vi "Inst_CNT90.vi"(8 "error in":errorcluster, 10 "All Message Queues in":T1, 11 "Prueba31 in":refnum<class "Prueba06.lvclass">) -> (0 "error out":errorcluster)   [LabVIEW 2019, in "Prueba06.lvclass"]
uses:
  Prueba06.lvclass
  QMH/Message Queue/All Message Queues.ctl
  QMH/Message Queue/Message Cluster.ctl
  Prueba06.lvclass/Prueba06.ctl
  <vilib>/Utility/error.llb/Error Cluster From Error Code.vi
  QMH/Message Queue/Enqueue Message (Single).vi
  <vilib>/ErrorRing/Error Ring.xnode
  QMH/Message Queue/Message Queue.lvlib
  Instrumento/CNT90/CNT90.lvclass
panel:
  out "All States":string[](array[string])
  out "Actual State":string
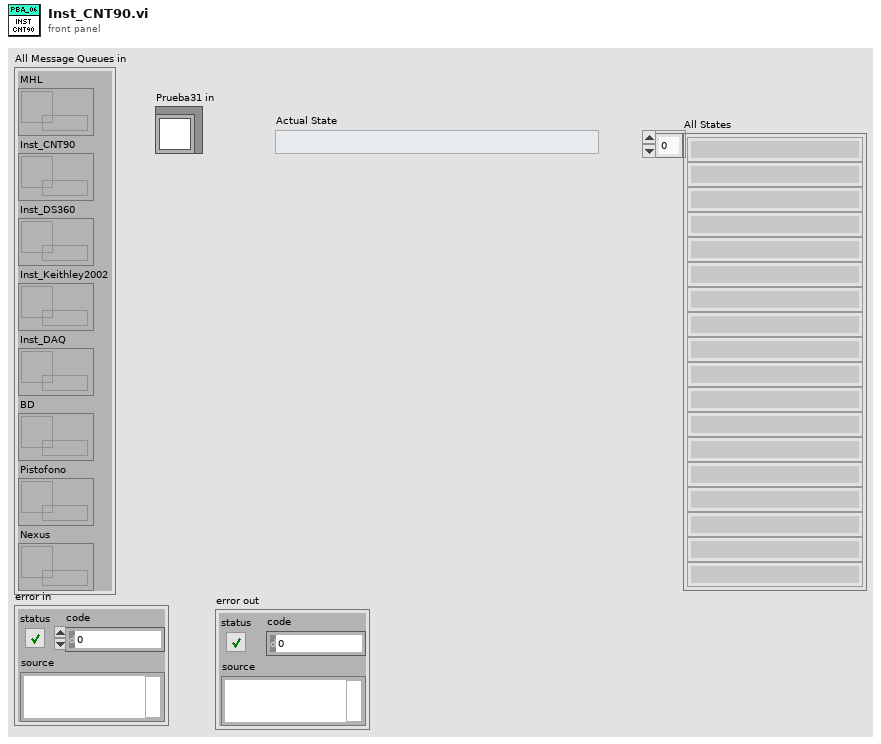
[diagram p1: front panel]
types:
  T1 = typedef "Message Queue.lvlib/All Message Queues.ctl" = cluster{"MHL":refnum<queue>, "Inst_CNT90":refnum<queue>, "Inst_DS360":refnum<queue>, "Inst_Keithley2002":refnum<queue>, "Inst_DAQ":refnum<queue>, "BD":refnum<queue>, "Pistofono":refnum<queue>, "Nexus":refnum<queue>}
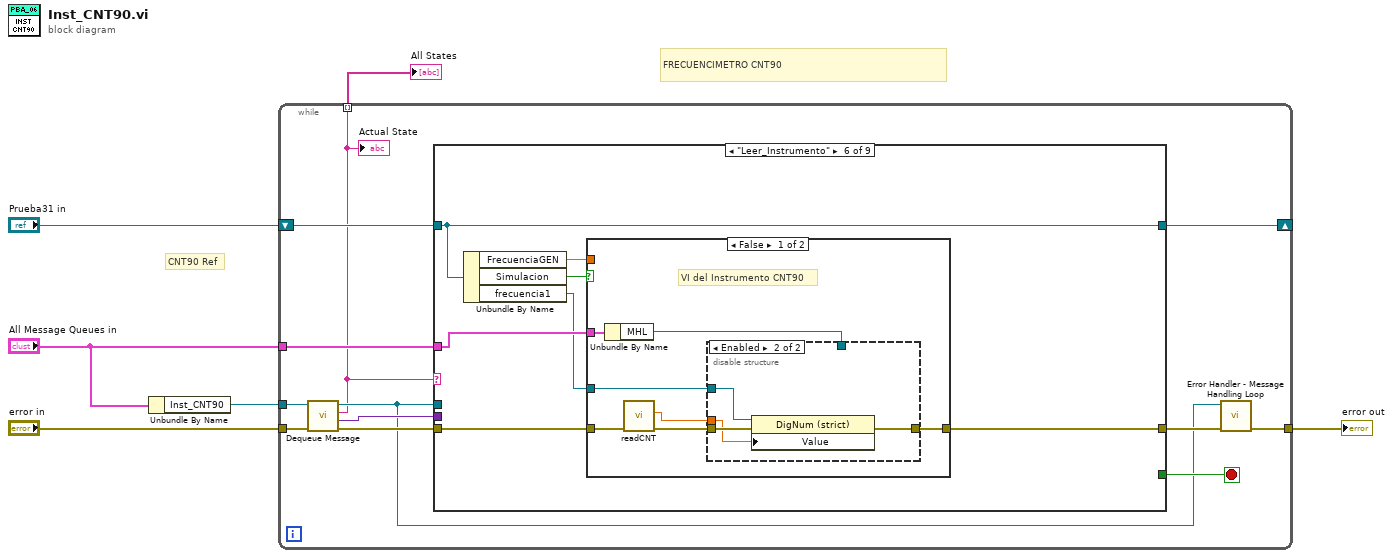
[diagram p0: block diagram]
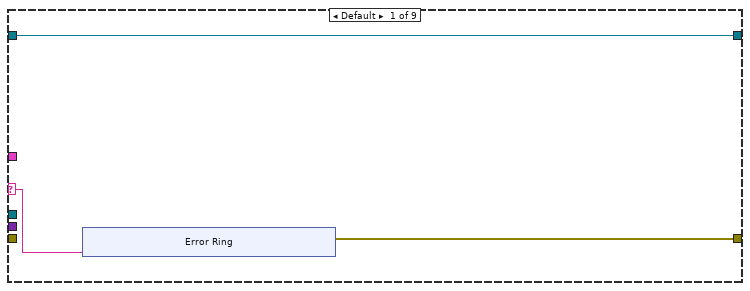
[diagram p2: hidden frame]
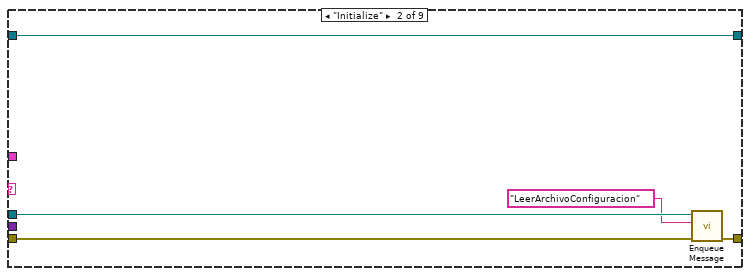
[diagram p3: hidden frame]
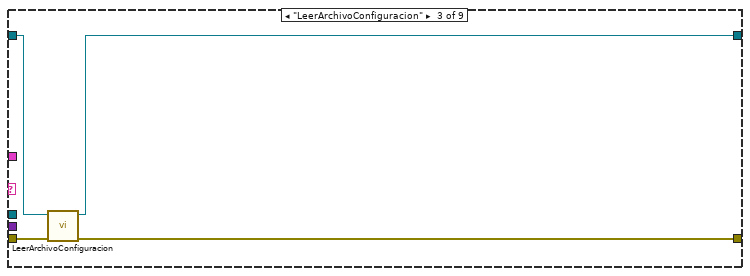
[diagram p4: hidden frame]
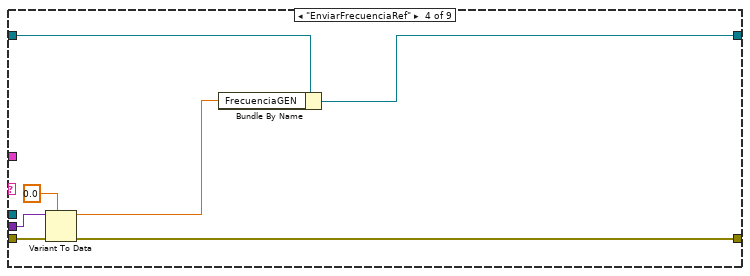
[diagram p5: hidden frame]
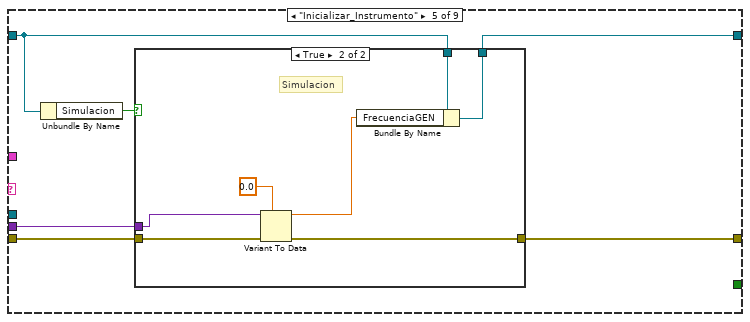
[diagram p6: hidden frame]
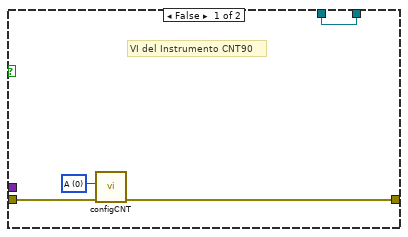
[diagram p7: hidden frame]
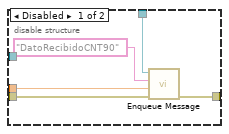
[diagram p8: hidden frame]
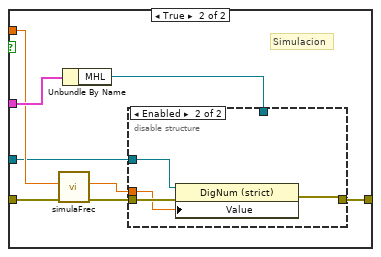
[diagram p9: hidden frame]
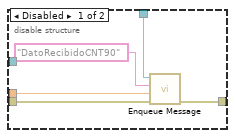
[diagram p10: hidden frame]
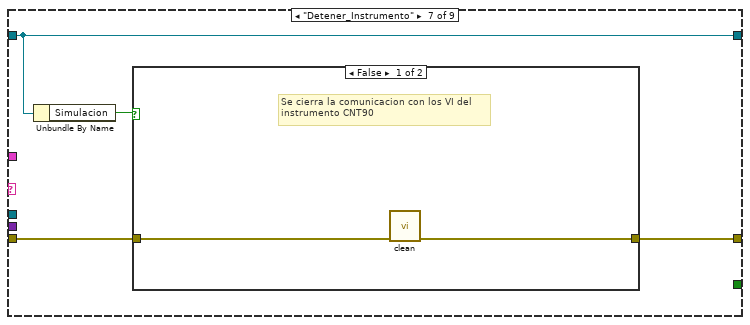
[diagram p11: hidden frame]
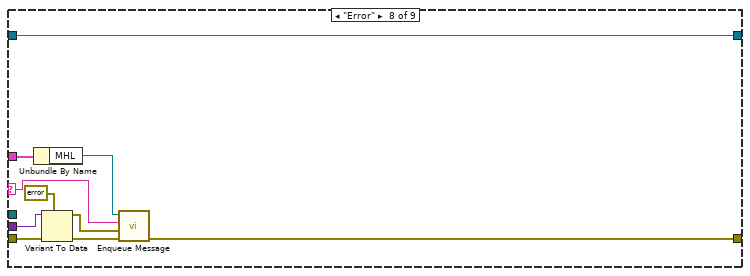
[diagram p13: hidden frame]
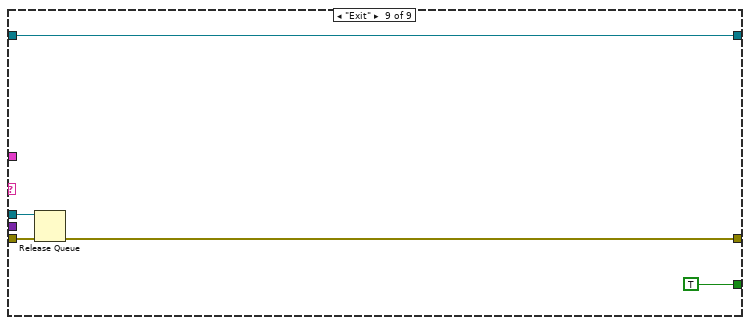
[diagram p14: hidden frame]
diagram:
  # "FRECUENCIMETRO CNT90"
  # "CNT90 Ref"
  n1 = Unbundle By Name("All Message Queues in") -> ("Inst_CNT90"=w4:refnum<queue>)
  n2 = while {
    tunnel: "error in" -> [w18]
    tunnel: w4 -> [w17]
    tunnel: "All Message Queues in" -> [w16]
    tunnel: [w9] -> w2
    shift-right: [w12] -> _
    shift-left: "Prueba31 in" -> [w15]
    tunnel: [w7] -> w1 mode=indexing
    stop <- w11 stop-if-true
    n3 = call "Dequeue Message.vi"("error in (no error)"=w18, "Message Queue"=w17) -> ("error out"=w13:errorcluster, "Message Data"=w14:variant, "Message"=w7:string, "dup Message Queue"=w8:refnum<queue>)  [unwired: 6 in]
    "Actual State" <- w7
    n4 = case shown="\"Leer_Instrumento\"" w7 {
      selector: w7 -> [w21 _ _ _ _ _ _ w113 _]
      tunnel: w16 -> [_ _ _ _ _ w64 _ w112 _]
      tunnel: w15 -> [w19 w33 w34 w39 w46 w66 w104 w110 w120]
      tunnel: w8 -> [_ w30 _ _ _ _ _ _ w122]
      tunnel: w14 -> [_ _ _ w42 w47 _ _ w116 _]
      tunnel: w13 -> [_ w31 w35 w43 w50 w68 w102 w117 w123]
      tunnel: [w20 w32 w37 w44 w48 w67 w105 w109 w119] -> w10
      tunnel: [w19 w33 w36 w40 w45 w66 w104 w110 w120] -> w12
      tunnel: [_ _ _ _ _ _ _ _ TRUE] -> w11
      frame Default {
        n5 = xnode "Error Ring"("parameter 0"=w21) -> ("error out"=w20:errorcluster)
      }
      frame "Initialize" {
        n6 = call-poly "Enqueue Message.vi"("error in (no error)"=w31, "Message"="LeerArchivoConfiguracion", "Message Queue"=w30) -> ("error out"=w32:errorcluster)  [unwired: 7 in, 1 out]
      }
      frame "LeerArchivoConfiguracion" {
        n7 = call "LeerArchivoConfiguracion.vi"("error in"=w35, "Prueba06 in"=w34) -> ("error out"=w37:errorcluster, "Prueba06 out"=w36:refnum<class "Prueba06.lvclass">)  [unwired: 8 in]
      }
      frame "EnviarFrecuenciaRef" {
        n8 = Variant To Data(error in=w43, type=0.0, Variant=w42) -> (data=w38:dbl, error out=w44:errorcluster)
        n9 = Bundle By Name(cluster=w39, "FrecuenciaGEN"=w38) -> (w40:refnum<class "Prueba06.lvclass">)
      }
      frame "Inicializar_Instrumento" {
        n10 = Unbundle By Name(w46) -> ("Simulacion"=w49:bool)
        n11 = case shown="True" w49 {
          tunnel: [w54 w60] -> w48
          tunnel: w50 -> [w53 w61]
          tunnel: w47 -> [_ w59]
          tunnel: w46 -> [w51 w57]
          tunnel: [w51 w56] -> w45
          frame False {
            w52 = 0 items=["A", "B"] ("Channel  1")
            # "VI del Instrumento CNT90"
            n12 = call "configCNT.vi"("error in (no error)"=w53, "Channel  1"=w52) -> ("error out"=w54:errorcluster)  [unwired: 8 in, 1 out]
          }
          frame True {
            # "Simulacion"
            n13 = Variant To Data(error in=w61, type=0.0, Variant=w59) -> (data=w55:dbl, error out=w60:errorcluster)
            n14 = Bundle By Name(cluster=w57, "FrecuenciaGEN"=w55) -> (w56:refnum<class "Prueba06.lvclass">)
          }
        }
      }
      frame "Leer_Instrumento" {
        n15 = Unbundle By Name(w66) -> ("FrecuenciaGEN"=w63:dbl, "Simulacion"=w65:bool, "frecuencia1"=w62:refnum<vi>)
        n16 = case shown="False" w65 {
          tunnel: [w72 w92] -> w67
          tunnel: w68 -> [w75 w89]
          tunnel: w64 -> [w71 w91]
          tunnel: w63 -> [_ w86]
          tunnel: w62 -> [w69 w85]
          frame False {
            # "VI del Instrumento CNT90"
            n17 = Unbundle By Name(w71) -> ("MHL"=w70:refnum<queue>)
            n18 = call "readCNT.vi"("error in (no error)"=w75) -> ("error out"=w73:errorcluster, "medicion"=w74:dbl)  [unwired: 8 in, 1 out]
            n19 = disable-structure shown="Enabled" {
              disable-tunnel: w74 -> [w80 w81]
              disable-tunnel: w73 -> [w78 w84]
              disable-tunnel: [w77 w83] -> w72
              disable-tunnel: w70 -> [w76 _]
              disable-tunnel: w69 -> [_ w82]
              frame Disabled {
                n20 = call-poly "Enqueue Message.vi"("error in (no error)"=w78, "Message Data"=w80, "Message"="DatoRecibidoCNT90", "Message Queue"=w76) -> ("error out"=w77:errorcluster)  [unwired: 6 in, 1 out]
              }
              frame Enabled {
                n21 = property class="DigNum (strict)"(reference=w82, error in=w84, "Value"=w81) -> (error out=w83:errorcluster)  [unwired: 1 out]
              }
            }
          }
          frame True {
            # "Simulacion"
            n22 = call "simulaFrec.vi"("error in (no error)"=w89, "frec in"=w86) -> ("error out"=w88:errorcluster, "frec out"=w87:dbl)  [unwired: 7 in, 1 out]
            n23 = Unbundle By Name(w91) -> ("MHL"=w90:refnum<queue>)
            n24 = disable-structure shown="Enabled" {
              disable-tunnel: [w96 w98] -> w92
              disable-tunnel: w90 -> [w95 _]
              disable-tunnel: w88 -> [w94 w101]
              disable-tunnel: w87 -> [w93 w100]
              disable-tunnel: w85 -> [_ w99]
              frame Disabled {
                n25 = call-poly "Enqueue Message.vi"("error in (no error)"=w94, "Message Data"=w93, "Message"="DatoRecibidoCNT90", "Message Queue"=w95) -> ("error out"=w96:errorcluster)  [unwired: 6 in, 1 out]
              }
              frame Enabled {
                n26 = property class="DigNum (strict)"(reference=w99, error in=w101, "Value"=w100) -> (error out=w98:errorcluster)  [unwired: 1 out]
              }
            }
          }
        }
      }
      frame "Detener_Instrumento" {
        n27 = Unbundle By Name(w104) -> ("Simulacion"=w103:bool)
        n28 = case shown="False" w103 {
          tunnel: [w107 w108] -> w105
          tunnel: w102 -> [w106 w108]
          frame False {
            # "Se cierra la comunicacion con los VI del\ninstrumento CNT90"
            n29 = call "clean.vi"("error in (no error)"=w106) -> ("error out"=w107:errorcluster)  [unwired: 9 in, 1 out]
          }
          frame True {
            # "Simulacion"
          }
        }
      }
      frame "Error" {
        n30 = Unbundle By Name(w112) -> ("MHL"=w111:refnum<queue>)
        n31 = Variant To Data(error in=w117, type=errorcluster {"status"=FALSE, "code"=0, "source"=""} ("error constant"), Variant=w116) -> (data=w114:errorcluster, error out=w115:errorcluster)
        n32 = call-poly "Enqueue Message.vi"("error in (no error)"=w115, "Message Data"=w114, "Message"=w113, "Message Queue"=w111) -> ("error out"=w109:errorcluster)  [unwired: 6 in, 1 out]
      }
      frame "Exit" {
        n33 = Release Queue(queue=w122, error in (no error)=w123) -> (error out=w119:errorcluster)  [unwired: 1 in, 2 out]
      }
    }
    n34 = call "Error Handler - Message Handling Loop.vi"("error in (no error)"=w10, "Message Queue"=w8) -> ("dup error in"=w9:errorcluster)  [unwired: 8 in, 1 out]
  }
  "error out" <- w2
  "All States" <- w1
